vi "Read Type.vi"(8 "error in (no error)":errorcluster, 11 "StopInstruction in":refnum<class "StopInstruction.lvclass">) -> (0 "error out":errorcluster, 2 "Type":string, 3 "StopInstruction out":refnum<class "StopInstruction.lvclass">)   [LabVIEW 2015, in "StopInstruction.lvclass"]
uses:
  StopInstruction.lvclass
  Instruction.lvclass
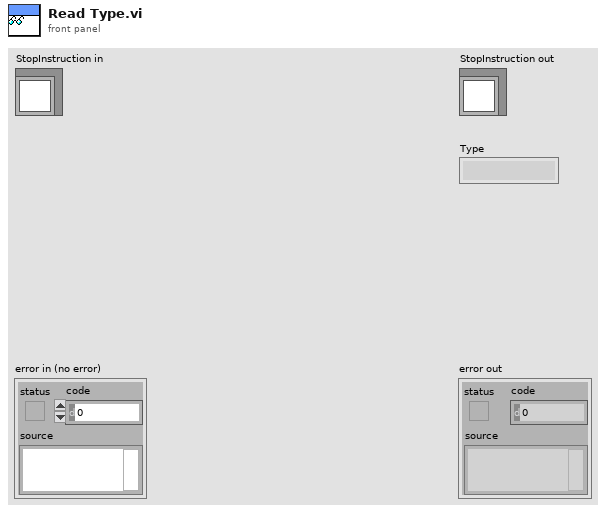
[diagram p1: front panel]
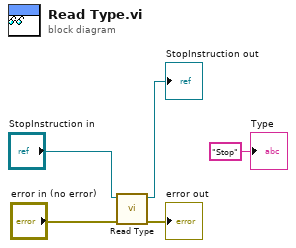
[diagram p0: block diagram]
diagram:
  n1 = call-parent "Read Type.vi"("error in (no error)"="error in (no error)", "Instruction in"="StopInstruction in") -> ("error out"=→"error out":errorcluster, "Instruction out"=→"StopInstruction out":refnum<class "StopInstruction.lvclass">)  [unwired: 7 in, 1 out]
  "Type" <- "Stop" ("Type")
